vi "get time stamp.vi"(8 "error in (no error)":errorcluster, 11 "Log File in":refnum<class "Log File.lvclass">) -> (0 "error out":errorcluster, 2 "time stamp":string, 3 "Log File out":refnum<class "Log File.lvclass">)   [LabVIEW 2018, in "Log File.lvclass"]
uses:
  Log File.lvclass
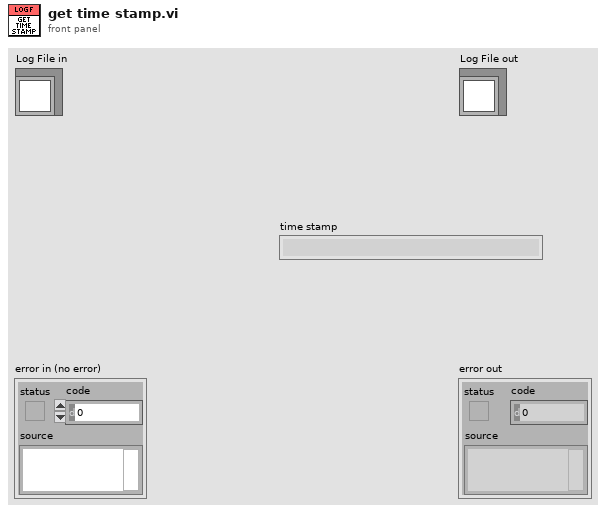
[diagram p1: front panel]
types:
  T1 = typedef "LVDateTimeRec.ctl" = cluster{"fractional second":dbl, "second":i32, "minute":i32, "hour":i32, "day of month":i32, "month":i32, "year":i32, "day of week":i32, "day of year":i32, "DST":i32}
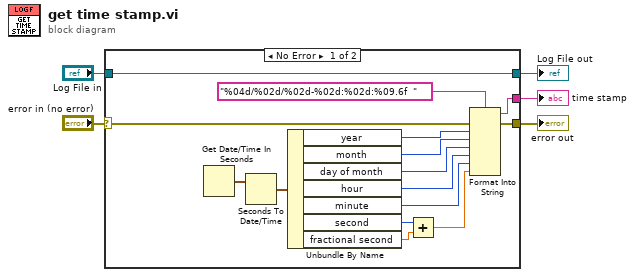
[diagram p0: block diagram]
diagram:
  n1 = case shown="No Error" "error in (no error)" {
    selector: "error in (no error)" -> [w8 w22]
    tunnel: [w6 w22] -> w4
    tunnel: [w16 w21] -> w2
    tunnel: "Log File in" -> [w16 w21]
    tunnel: [w7 _] -> w1
    frame No Error {
      n2 = Get Date/Time In Seconds() -> (seconds since 1Jan1904=w20:timestamp)
      n3 = Seconds To Date/Time(time stamp (now)=w20) -> (date time rec=w19:T1)  [unwired: 1 in]
      n4 = Unbundle By Name(w19) -> ("year"=w15:i32, "month"=w14:i32, "day of month"=w13:i32, "hour"=w12:i32, "minute"=w11:i32, "second"=w18:i32, "fractional second"=w17:dbl)
      n5 = Add(x=w18, y=w17) -> (x+y=w10:dbl)
      n6 = Format Into String(format string="%04d/%02d/%02d-%02d:%02d:%09.6f  ", error in=w8, w15, w14, w13, w12, w11, w10) -> (resulting string=w7:string, error out=w6:errorcluster)  [unwired: 1 in]
    }
    frame Error {
    }
  }
  "error out" <- w4
  "Log File out" <- w2
  "time stamp" <- w1
